vi "bias_on_off_ext.vi"() -> ()   [LabVIEW 2011]
panel:
  in  "Frequency":dbl
  out "STATE":bool
  in  "STOP":bool
  out "error out":errorcluster
  out "VISA Out":refnum<visa-resource-name>
  in  "VISA In":refnum<visa-resource-name>
  in  "error in (no error)":errorcluster
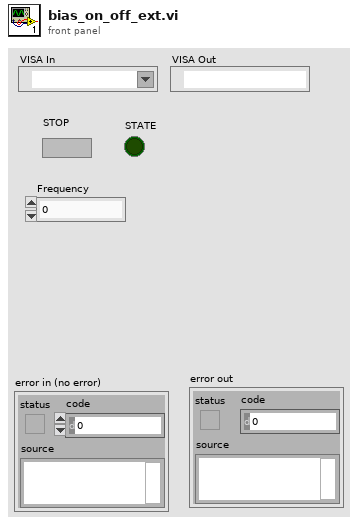
[diagram p1: front panel]
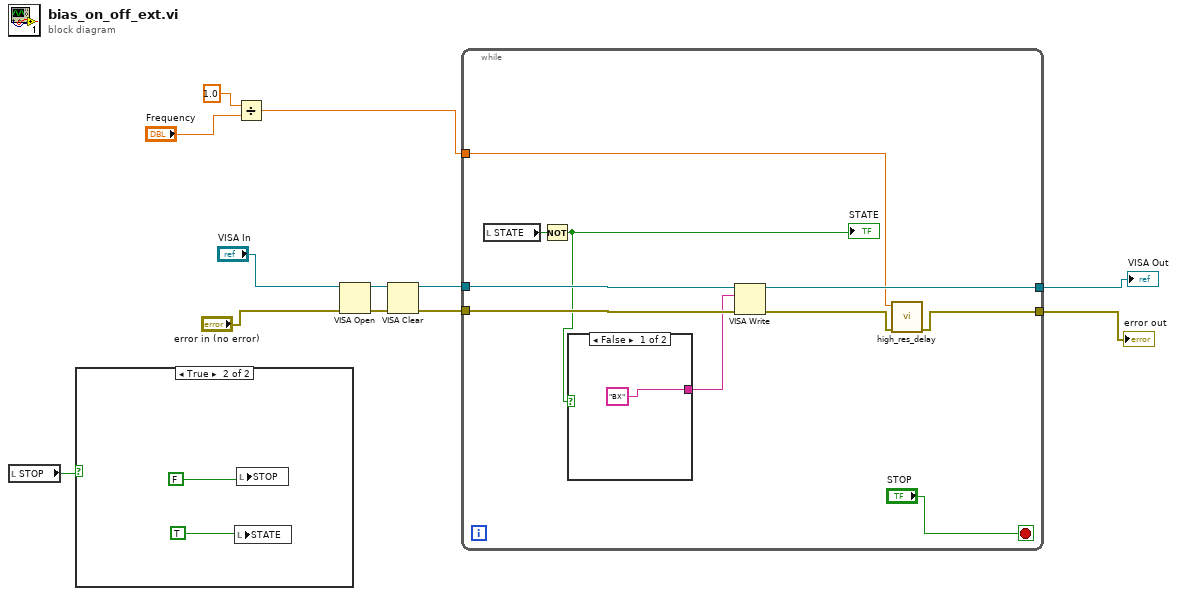
[diagram p0: block diagram]
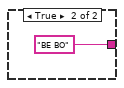
[diagram p3: hidden frame]
diagram:
  n1 = local read "STOP"() -> (w8:bool)
  n2 = case shown="True" w8 {
    frame False {
    }
    frame True {
      n3 = local write "STATE"(TRUE) -> ()
      n4 = local write "STOP"(FALSE) -> ()
    }
  }
  n5 = Divide(x=1.0, y="Frequency") -> (x/y=w1:dbl)
  n6 = VISA Open(error in (no error)="error in (no error)", VISA resource name="VISA In") -> (VISA resource name=w11:refnum<visa-resource-name>, error out=w12:errorcluster)  [unwired: 3 in]
  n7 = VISA Clear(VISA resource name=w11, error in (no error)=w12) -> (VISA resource name out=w10:refnum<visa-resource-name>, error out=w9:errorcluster)
  n8 = while {
    tunnel: w10 -> [w24]
    tunnel: w9 -> [w23]
    tunnel: [w19] -> w5
    tunnel: [w18] -> w4
    tunnel: w1 -> [w16]
    stop <- "STOP" stop-if-true
    n9 = local read "STATE"() -> (w21:bool)
    n10 = Not(x=w21) -> (.not. x?=w15:bool)
    "STATE" <- w15
    n11 = case shown="False" w15 {
      tunnel: ["BX" "BE BO"] -> w20
      frame False {
      }
      frame True {
      }
    }
    n12 = VISA Write(VISA resource name=w24, write buffer=w20, error in (no error)=w23) -> (VISA resource name out=w19:refnum<visa-resource-name>, error out=w17:errorcluster)  [unwired: 1 out]
    n13 = call "high_res_delay.vi"("error in (no error)"=w17, "Delay (sec)"=w16) -> ("error out"=w18:errorcluster)  [unwired: 9 in]
  }
  "VISA Out" <- w5
  "error out" <- w4
